vi "Write Random_B Msg.vi"(10 "B_Actor.lvlib:Random_B Msg.lvclass":refnum<class "Random_B Msg.lvclass">, 11 "B_Actor in":refnum<class "B_Actor.lvclass">) -> (3 "B_Actor out":refnum<class "B_Actor.lvclass">)   [LabVIEW 2025, in "B_Actor.lvlib" / "B_Actor.lvclass"]
uses:
  B_Actor.lvclass
  B_Actor Messages/Random_B Msg/Random_B Msg.lvclass
  B_Actor.lvclass/B_Actor.ctl
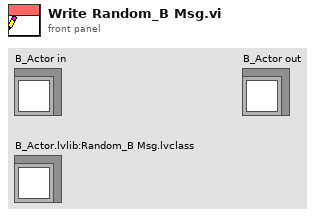
[diagram p1: front panel]
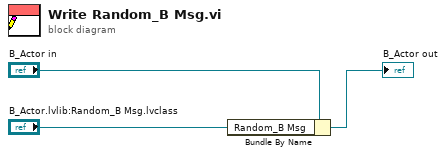
[diagram p0: block diagram]
diagram:
  n1 = Bundle By Name(cluster="B_Actor in", "Random_B Msg"="B_Actor.lvlib:Random_B Msg.lvclass") -> (→"B_Actor out":refnum<class "B_Actor.lvclass">)
